vi "observacao.vi"() -> ()   [LabVIEW 2018, in "Shared_160.lvlib"] (continued)
                n2314 = call "TickTimeout.vi"("msInicial"=w2963, "msTimeout"=u32 2000) -> ("msTick"=w2966:u32, "Timeout"=w2965:bool)  [unwired: 1 out]
                n2315 = case shown="True" w2965 {
                  tunnel: w2966 -> [_ w2967]
                  frame False {
                  }
                  frame True {
                    n2316 = global write "Global_Telescopio.vi" "RevCupTO"(w2967) -> ()
                    n2317 = local write "StatDome"("Not Ready" ("Status")) -> ()
                  }
                }
              }
              frame Enabled {
              }
            }
            n2318 = global read "Global_Telescopio.vi" "Senha LEAF"() -> (w2897:string)
            n2319 = call "Bit Status CUP.vi"("NomeStatus"=w2903) -> ("StatBit"=→"trapeiraFechada":bool)
            n2320 = call "Bit Status CUP.vi"("NomeStatus"=w2904) -> ("StatBit"=w2894:bool)
            "trapeiraMovendo" <- w2894
            n2321 = call "Bit Status CUP.vi"("NomeStatus"=w2902) -> ("StatBit"=→"trapeiraAberta":bool)
            n2322 = Not(x=w2894) -> (.not. x?=w2895:bool)
            n2323 = property on="Setup, Pointing & Guiding" class="TabCtl (strict)"("Page Selector Visible"=w2895) -> ()  [unwired: 2 in, 2 out]
            n2324 = Match Pattern(string="OpenShutterPassword", regular expression=w2897) -> (offset past match=w2899:i32)  [unwired: 1 in, 3 out]
            n2325 = Greater Or Equal To 0?(x=w2899) -> (x >= 0?=w2896:bool)
            n2326 = global read "Global_Telescopio.vi" "Telescopio"() -> (w2909:bool)
            n2327 = local read "StatDome"() -> (w2915:string)
            n2328 = Select(t=1, s=w2909, f=2) -> (s? t:f=w2907:i32)
            n2329 = event shown="[3] \"BtShutterOpen\": Value Change" {
              selector: _ -> [_ _ _ _ _ _ _ _]
              dyn-events: _ -> [_ _ _ _ _ _ _ _]
              timeout: 10 -> [_ _ _ _ _ _ _ _]
              tunnel: [FALSE ("NewVal") w3015 w3028 FALSE ("NewVal") FALSE ("NewVal") _ _ _] -> w2913
              tunnel: w2907 -> [_ w3014 _ _ _ _ _ _]
              tunnel: w2896 -> [_ _ _ w3035 _ _ _ _]
              event Timeout {
                n2330 = event-data() -> ()  [unwired: 1 in, 2 out]
              }
              event "BtDomeGO": Value Change {
                n2331 = event-data() -> ("NewVal"=w3016:bool)  [unwired: 1 in, 5 out]
                n2332 = local read "StatDome"() -> (w3019:string)
                n2333 = Equal?(x=w3019, y="Stopped" ("Status")) -> (x = y?=w3017:bool)
                n2334 = And(x=w3016, y=w3017) -> (x .and. y?=w3015:bool)
                n2335 = case shown="True" w3015 {
                  tunnel: w3014 -> [_ w3023]
                  frame False {
                  }
                  frame True {
                    # "20240820"
                    n2336 = local read "DomeNewPos"() -> (w3020:i32)
                    n2337 = Multiply(x=w3020, y=w3023) -> (x*y=w3021:i32)
                    n2338 = call "Checa destino cupula.vi"("Target"=w3021) -> ("moverCup"=w3022:bool)  [unwired: 6 in, 2 out]
                    n2339 = case shown="True" w3022 {
                      tunnel: w3021 -> [_ w3026]
                      frame False {
                      }
                      frame True {
                        # "Desabilita todas Abas"
                        n2340 = local write "DestCUP"(w3026) -> ()
                        n2341 = local write "DOME"(FALSE) -> ()
                        n2342 = property on="Setup, Pointing & Guiding" class="TabCtl (strict)"("Page Selector Visible"=FALSE) -> ()  [unwired: 2 in, 2 out]
                        n2343 = local write "StatDome"("Not Ready" ("Status")) -> ()
                      }
                    }
                  }
                }
              }
              event "BtDomeSTOP": Value Change {
                n2344 = event-data() -> ("NewVal"=w3028:bool)  [unwired: 1 in, 5 out]
                n2345 = case shown="True" w3028 {
                  frame False {
                  }
                  frame True {
                    n2346 = local read "StatDome"() -> (w3029:string)
                    n2347 = case shown="\"Moving\", Default" w3029 {
                      frame "Stopped" {
                      }
                      frame "Moving", Default {
                        w3030 = u16 4 items=["ZERO", "AH", "DEC", "TUBO", "CUP"] ("Controlador")
                        n2348 = local write "StatDome"("Stopping" ("Status")) -> ()
                        n2349 = call "Monta Comando.vi"("Comando"="PARAR", "Dispositivo"="PROG", "Controlador"=w3030) -> ()  [unwired: 2 in, 5 out]
                      }
                      frame "Not Ready" {
                        n2350 = local write "StatDome"("Stopped" ("Status")) -> ()
                      }
                    }
                  }
                }
              }
              event "BtShutterOpen": Value Change {
                # "20250912)"
                n2351 = event-data() -> ("NewVal"=w3038:bool)  [unwired: 1 in, 5 out]
                n2352 = local write "OpenShutterPassword"("") -> ()
                n2353 = And(x=w3038, y=w3035) -> (x .and. y?=w3037:bool)
                n2354 = case shown="True" w3037 {
                  frame False {
                  }
                  frame True {
                    w3040 = FALSE ("WeakSel")
                    w3044 = T5."Enabled" ("Disabled")
                    n2355 = property on="Weak" class="Bool (strict)"("Disabled"=w3044) -> ()  [unwired: 2 in, 2 out]
                    n2356 = local write "Weak"(w3040) -> ()
                    n2357 = local write "WeakSel"(w3040) -> ()
                    n2358 = property on="Medium" class="Bool (strict)"("Disabled"=w3044) -> ()  [unwired: 2 in, 2 out]
                    n2359 = local write "Medium"(w3040) -> ()
                    n2360 = local write "MediumSel"(w3040) -> ()
                    n2361 = call "Log_Shutter.vi"("command"=" ", "domeState"="OPEN " ("command"), "pathLogDomeFile"="C:\\TCS\\LOG\\SHUTTER\\SHUTTER.TXT" ("pathLogFocoString")) -> ()  [unwired: 6 in]
                    n2362 = property on="Strong" class="Bool (strict)"("Disabled"=w3044) -> ()  [unwired: 2 in, 2 out]
                    n2363 = local write "Strong"(w3040) -> ()
                    n2364 = local write "StrongSel"(w3040) -> ()
                    n2365 = stacked-sequence {
                      frame #0 {
                        w3046 = u16 4 items=["ZERO", "AH", "DEC", "TUBO", "CUP"] ("Controlador")
                        n2366 = call "Monta Comando.vi"("Comando"="DESLIGAR", "Dispositivo"="FLAT_WEAK", "Controlador"=w3046) -> ()  [unwired: 2 in, 5 out]
                      }
                      frame #1 {
                        w3049 = u16 4 items=["ZERO", "AH", "DEC", "TUBO", "CUP"] ("Controlador")
                        n2367 = call "Monta Comando.vi"("Comando"="DESLIGAR", "Dispositivo"="FLAT_LO", "Controlador"=w3049) -> ()  [unwired: 2 in, 5 out]
                      }
                      frame #2 {
                        w3052 = u16 4 items=["ZERO", "AH", "DEC", "TUBO", "CUP"] ("Controlador")
                        n2368 = call "Monta Comando.vi"("Comando"="DESLIGAR", "Dispositivo"="FLAT_HI", "Controlador"=w3052) -> ()  [unwired: 2 in, 5 out]
                      }
                      frame #3 {
                        w3054 = u16 4 items=["ZERO", "AH", "DEC", "TUBO", "CUP"] ("Controlador")
                        n2369 = call "Monta Comando.vi"("Comando"="DESLIGAR", "Dispositivo"="FLAT_COUDE", "Controlador"=w3054) -> ()  [unwired: 2 in, 5 out]
                      }
                      frame #4 {
                        w3057 = u16 4 items=["ZERO", "AH", "DEC", "TUBO", "CUP"] ("Controlador")
                        n2370 = call "Monta Comando.vi"("Comando"="ABRIR", "Dispositivo"="TRAPEIRA" ("Comando"), "Controlador"=w3057) -> ()  [unwired: 2 in, 5 out]
                      }
                    }
                    n2371 = property on="Coude" class="Bool (strict)"("DisabledEnum"=w3044) -> ()  [unwired: 2 in, 2 out]
                    n2372 = local write "Coude"(w3040) -> ()
                    n2373 = local write "CoudeSel"(w3040) -> ()
                  }
                }
              }
              event "BtShutterClose": Value Change {
                # "20250912)"
                n2374 = event-data() -> ("NewVal"=w3062:bool)  [unwired: 1 in, 5 out]
                n2375 = local write "OpenShutterPassword"("") -> ()
                n2376 = case shown="True" w3062 {
                  frame False {
                  }
                  frame True {
                    w3064 = u16 4 items=["ZERO", "AH", "DEC", "TUBO", "CUP"] ("Controlador")
                    # "Escreve no LOG o estado do shutter"
                    n2377 = call "Log_Shutter.vi"("command"=" ", "domeState"="CLOSED " ("command"), "pathLogDomeFile"="C:\\TCS\\LOG\\SHUTTER\\SHUTTER.TXT" ("pathLogFocoString")) -> ()  [unwired: 6 in]
                    n2378 = call "Monta Comando.vi"("Comando"="FECHAR", "Dispositivo"="TRAPEIRA" ("Comando"), "Controlador"=w3064) -> ()  [unwired: 2 in, 5 out]
                  }
                }
              }
              event "BtParavUp": Value Change {
                n2379 = event-data() -> ("NewVal"=w3069:bool)  [unwired: 1 in, 5 out]
                n2380 = case shown="True" w3069 {
                  frame False {
                  }
                  frame True {
                    w3072 = u16 4 items=["ZERO", "AH", "DEC", "TUBO", "CUP"] ("Controlador")
                    n2381 = call "Monta Comando.vi"("Comando"="SUBIR", "Dispositivo"="PARAVENTO" ("Comando"), "Controlador"=w3072) -> ()  [unwired: 2 in, 5 out]
                  }
                }
              }
              event "BtParavDown": Value Change {
                n2382 = event-data() -> ("NewVal"=w3073:bool)  [unwired: 1 in, 5 out]
                n2383 = case shown="True" w3073 {
                  frame False {
                  }
                  frame True {
                    w3076 = u16 4 items=["ZERO", "AH", "DEC", "TUBO", "CUP"] ("Controlador")
                    n2384 = call "Monta Comando.vi"("Comando"="DESCER", "Dispositivo"="PARAVENTO" ("Comando"), "Controlador"=w3076) -> ()  [unwired: 2 in, 5 out]
                  }
                }
              }
              event "BtParavStop": Value Change {
                n2385 = event-data() -> ("NewVal"=w3077:bool)  [unwired: 1 in, 5 out]
                n2386 = case shown="True" w3077 {
                  frame False {
                  }
                  frame True {
                    w3080 = u16 4 items=["ZERO", "AH", "DEC", "TUBO", "CUP"] ("Controlador")
                    n2387 = call "Monta Comando.vi"("Comando"="PARAR", "Dispositivo"="PARAVENTO" ("Comando"), "Controlador"=w3080) -> ()  [unwired: 2 in, 5 out]
                  }
                }
              }
            }
            n2388 = call "Bit Status CUP.vi"("NomeStatus"=w2914) -> ("StatBit"=w2912:bool)
            n2389 = global read "Global_Telescopio.vi" "PosCUP"() -> (w2911:i16)
            n2390 = case shown="\"Not Ready\"" w2915 {
              tunnel: w2912 -> [_ _ w3004 w3010]
              tunnel: w2913 -> [_ _ _ _]
              frame "", Default {
              }
              frame "Not Ready" {
                n2391 = local read "DestCUP"() -> (w2990:i16)
                n2392 = global read "Global_Telescopio.vi" "PosCUP"() -> (w2992:i16)
                n2393 = call "TickTimeout.vi"() -> ("msTick"=w2993:u32)  [unwired: 2 in, 2 out]
                n2394 = call "Checa destino cupula.vi"("Target"=w2990) -> ("moverCup"=w2989:bool, "angTarget"=w2991:string)  [unwired: 6 in, 1 out]
                n2395 = case shown="True" w2989 {
                  tunnel: w2993 -> [_ w2999]
                  tunnel: w2992 -> [_ w2998]
                  tunnel: w2991 -> [_ w2997]
                  tunnel: w2990 -> [_ w2996]
                  frame False {
                    n2396 = local write "StatDome"("Stopping" ("Status")) -> ()
                  }
                  frame True {
                    w3003 = u16 4 items=["ZERO", "AH", "DEC", "TUBO", "CUP"] ("Controlador")
                    # "20240820"
                    n2397 = global write "Global_Telescopio.vi" "RevCupTO"(w2999) -> ()
                    n2398 = local write "TargetCup"(w2997) -> ()
                    n2399 = global write "Global_Telescopio.vi" "CupStartPos"(w2998) -> ()
                    n2400 = Number To Decimal String(number=w2996) -> (decimal integer string=w3000:string)  [unwired: 1 in]
                    n2401 = local write "StatDome"("Moving" ("Status")) -> ()
                    n2402 = call "Monta Comando.vi"("Set Point"=w3000, "Comando"="MOVER", "Dispositivo"="DOMO" ("Comando"), "Controlador"=w3003) -> ()  [unwired: 1 in, 5 out]
                  }
                }
              }
              frame "Moving" {
                n2403 = case shown="False" w3004 {
                  frame False {
                    n2404 = local read "DestCUP"() -> (w3009:i16)
                    n2405 = call "Checa destino cupula.vi"("Target"=w3009) -> ("moverCup"=w3008:bool)  [unwired: 6 in, 2 out]
                    n2406 = Select(t="Not Ready" ("Comando"), s=w3008, f="Stopping" ("Comando")) -> (s? t:f=w3007:string)
                    n2407 = local write "StatDome"(w3007) -> ()
                  }
                  frame True {
                  }
                }
              }
              frame "Stopping" {
                n2408 = case shown="False" w3010 {
                  frame False {
                    # "Reabilita Abas"
                    n2409 = property on="Setup, Pointing & Guiding" class="TabCtl (strict)"("Page Selector Visible"=TRUE) -> ()  [unwired: 2 in, 2 out]
                    n2410 = local write "StatDome"("Stopped" ("Status")) -> ()
                  }
                  frame True {
                  }
                }
              }
            }
            n2411 = Divide(x=w2911, y=w2907) -> (x/y=w2918:dbl)
            n2412 = To Word Integer(number=w2918) -> (16bit integer=→"AngCup":i16)
            n2413 = event shown="[4] \"CW\": Mouse Up" {
              selector: _ -> [_ _ _ _ _]
              dyn-events: _ -> [_ _ _ _ _]
              timeout: 100 -> [_ _ _ _ _]
              event Timeout {
                n2414 = event-data() -> ()  [unwired: 1 in, 2 out]
              }
              event "CCW": Mouse Down {
                w2969 = "GIRAR_CCW" ("Comando")
                w2970 = u16 4 items=["ZERO", "AH", "DEC", "TUBO", "CUP"] ("Controlador")
                # "Envia o comando GIRAR"
                n2415 = event-data() -> ()  [unwired: 1 in, 7 out]
                n2416 = local write "Command"(w2969) -> ()
                n2417 = call "Monta Comando.vi"("Comando"=w2969, "Dispositivo"="DOMO" ("Comando"), "Controlador"=w2970) -> ()  [unwired: 2 in, 5 out]
              }
              event "CCW": Mouse Up {
                n2418 = event-data() -> ()  [unwired: 1 in, 7 out]
                n2419 = stacked-sequence {
                  frame #0 {
                    w2972 = "PARAR" ("Comando")
                    w2973 = u16 4 items=["ZERO", "AH", "DEC", "TUBO", "CUP"] ("Controlador")
                    # "Envia o comando PARAR"
                    n2420 = local write "Command"(w2972) -> ()
                    n2421 = call "Monta Comando.vi"("Comando"=w2972, "Dispositivo"="DOMO" ("Comando"), "Controlador"=w2973) -> ()  [unwired: 2 in, 5 out]
                  }
                  frame #1 {
                    n2422 = Wait (ms)(milliseconds to wait=u32 100) -> ()  [unwired: 1 out]
                  }
                  frame #2 {
                    w2976 = "PARAR" ("Comando")
                    w2977 = u16 4 items=["ZERO", "AH", "DEC", "TUBO", "CUP"] ("Controlador")
                    # "Envia o comando PARAR"
                    n2423 = local write "Command"(w2976) -> ()
                    n2424 = call "Monta Comando.vi"("Comando"=w2976, "Dispositivo"="DOMO" ("Comando"), "Controlador"=w2977) -> ()  [unwired: 2 in, 5 out]
                  }
                }
              }
              event "CW": Mouse Down {
                w2979 = "GIRAR_CW" ("Comando")
                w2980 = u16 4 items=["ZERO", "AH", "DEC", "TUBO", "CUP"] ("Controlador")
                # "Envia o comando GIRAR"
                n2425 = event-data() -> ()  [unwired: 1 in, 7 out]
                n2426 = local write "Command"(w2979) -> ()
                n2427 = call "Monta Comando.vi"("Comando"=w2979, "Dispositivo"="DOMO" ("Comando"), "Controlador"=w2980) -> ()  [unwired: 2 in, 5 out]
              }
              event "CW": Mouse Up {
                n2428 = event-data() -> ()  [unwired: 1 in, 7 out]
                n2429 = stacked-sequence {
                  frame #0 {
                    w2982 = "PARAR" ("Comando")
                    w2983 = u16 4 items=["ZERO", "AH", "DEC", "TUBO", "CUP"] ("Controlador")
                    # "Envia o comando PARAR"
                    n2430 = local write "Command"(w2982) -> ()
                    n2431 = call "Monta Comando.vi"("Comando"=w2982, "Dispositivo"="DOMO" ("Comando"), "Controlador"=w2983) -> ()  [unwired: 2 in, 5 out]
                  }
                  frame #1 {
                    n2432 = Wait (ms)(milliseconds to wait=u32 100) -> ()  [unwired: 1 out]
                  }
                  frame #2 {
                    w2986 = "PARAR" ("Comando")
                    w2987 = u16 4 items=["ZERO", "AH", "DEC", "TUBO", "CUP"] ("Controlador")
                    # "Envia o comando PARAR"
                    n2433 = local write "Command"(w2986) -> ()
                    n2434 = call "Monta Comando.vi"("Comando"=w2986, "Dispositivo"="DOMO" ("Comando"), "Controlador"=w2987) -> ()  [unwired: 2 in, 5 out]
                  }
                }
              }
            }
            "Command" <- "" ("Command")
          }
          frame "UTILS " {
            n2435 = stacked-sequence {
              frame #0 {
                # "Acionamento das Abas do\nEspelho\n\nComandos sempre precedidos\nde ESPAÇO\n\nTUBO TAMPAS ESCREVER = 80 80\n\nLigar power geral       08 08\nDesligar power geral  08 00\nLigar System              10 10\nDesligar System         10 00\nPassar para Remoto  20 20\nPassar para Local      20 00\nSel. device central     40 40\nSel. device bowl         40 00\nAction open                80 80\nAction close                80 00"
                n2436 = event shown="[1] \"MODE\": Value Change" {
                  selector: _ -> [_ _ _]
                  dyn-events: _ -> [_ _ _]
                  timeout: 10 -> [_ _ _]
                  event Timeout {
                    n2437 = event-data() -> ()  [unwired: 1 in, 2 out]
                  }
                  event "MODE": Value Change {
                    n2438 = event-data() -> ("NewVal"=w3095:bool)  [unwired: 1 in, 5 out]
                    "LED MODE" <- w3095
                    n2439 = case shown="False" w3095 {
                      frame False {
                        w3100 = u16 3 items=["ZERO", "AH", "DEC", "TUBO", "CUP"] ("Controlador")
                        # "DESABILITA"
                        # "APENAS PASSANDO COMANDO PARA MANETE"
                        # "MODE E GERAL = 0"
                        # "MODE HADSET"
                        n2440 = call "Monta Comando.vi"("Set Point"=" F8 90", "Comando"="ESCREVER", "Dispositivo"="TAMPAS" ("Comando"), "Controlador"=w3100) -> ()  [unwired: 1 in, 5 out]
                        n2441 = property on="ACTION" class="Bool (strict)"("Disabled"=u8 2) -> ()  [unwired: 2 in, 2 out]
                      }
                      frame True {
                        w3105 = u16 3 items=["ZERO", "AH", "DEC", "TUBO", "CUP"] ("Controlador")
                        # "HABILITA"
                        # "APENAS PASSANDO COMOANDO PARA TCSPD"
                        # "MODE E GERAL = 1"
                        # "MODE TCSPD"
                        n2442 = call "Monta Comando.vi"("Set Point"=" 48 48", "Comando"="ESCREVER", "Dispositivo"="TAMPAS" ("Comando"), "Controlador"=w3105) -> ()  [unwired: 1 in, 5 out]
                        n2443 = property on="ACTION" class="Bool (strict)"("Disabled"=u8 0) -> ()  [unwired: 2 in, 2 out]
                      }
                    }
                  }
                  event "ACTION": Value Change {
                    n2444 = event-data() -> ("NewVal"=w3106:bool)  [unwired: 1 in, 5 out]
                    n2445 = case shown="False" w3106 {
                      frame False {
                        # "FECHAR"
                        n2446 = local write "ESTADO FECHAR"("INICIO" ("ESTADO ABRIR")) -> ()
                        n2447 = local write "ESTADO ABRIR"("REPOUSO" ("ESTADO ABRIR")) -> ()
                      }
                      frame True {
                        # "ABRIR"
                        n2448 = local write "ESTADO FECHAR"("REPOUSO" ("ESTADO ABRIR")) -> ()
                        n2449 = local write "ESTADO ABRIR"("INICIO" ("ESTADO ABRIR")) -> ()
                      }
                    }
                  }
                }
                n2450 = Tick Count (ms)() -> (millisecond timer value=w3086:u32)
                n2451 = Greater Or Equal?(x=w3086, y="TIMER TICK") -> (x >= y?=w3082:bool)
                n2452 = And(x=w3082, y=FALSE) -> (x .and. y?=w3083:bool)
                n2453 = case shown="True" w3083 {
                  frame False {
                  }
                  frame True {
                    w3119 = u16 3 items=["ZERO", "AH", "DEC", "TUBO", "CUP", "CASS", "COUDE"] ("Controlador")
                    # "2 SEGUNDOS"
                    n2454 = Tick Count (ms)() -> (millisecond timer value=w3116:u32)
                    n2455 = Add(x=w3116, y=u32 10000) -> (x+y=w3114:u32)
                    n2456 = call "Status_das_Tampas.vi"("Controlador"=w3119, "DISPOSITIVO"="TAMPAS", "Comando"="LER") -> ("Fechado/Aberto"=w3113:bool, "Dispositivo Bacia/Centar"=w3112:bool)  [unwired: 6 in, 5 out]
                    n2457 = local write "TIMER TICK"(w3114) -> ()
                    n2458 = Not(x=w3113) -> (.not. x?=w3111:bool)
                    n2459 = And(x=w3111, y=w3112) -> ()  [unwired: 1 out]
                  }
                }
                n2460 = event shown="[4] \"FLAT-FIELD\": Value Change" {
                  selector: _ -> [_ _ _ _ _ _]
                  dyn-events: _ -> [_ _ _ _ _ _]
                  timeout: 10 -> [_ _ _ _ _ _]
                  event Timeout {
                    n2461 = event-data() -> ()  [unwired: 1 in, 2 out]
                  }
                  event "BtUtilPark": Value Change {
                    n2462 = event-data() -> ("NewVal"=w3120:bool)  [unwired: 1 in, 5 out]
                    n2463 = case shown="True" w3120 {
                      frame False {
                      }
                      frame True {
                        w3123 = u16 4 items=["ZERO", "AH", "DEC", "TUBO", "CUP"] ("Controlador")
                        w3124 = FALSE ("MOUNT")
                        w3127 = 0 ("M_AH")
                        w3128 = u8 2 ("Disabled")
                        w3125 = FALSE ("Page Selector Visible")
                        w3132 = 1 ("M_AH")
                        # "Carrega Parâmetros da Configuração"
                        # "Seta Máq GO"
                        # "Desabilita todas Abas"
                        # "DESABILITA TODOS"
                        n2464 = local write "DOME"(w3125) -> ()
                        n2465 = property on="Setup, Pointing & Guiding" class="TabCtl (strict)"("Page Selector Visible"=w3125) -> ()  [unwired: 2 in, 2 out]
                        n2466 = local write "statAH"(w3127) -> ()
                        n2467 = local write "statCUP"(w3127) -> ()
                        n2468 = local write "statDEC"(w3127) -> ()
                        n2469 = local write "M_DEC"(w3132) -> ()
                        n2470 = local write "M_AH"(w3132) -> ()
                        n2471 = local write "M_CUP"(w3132) -> ()
                        n2472 = global read "Global_Telescopio.vi" "DestDEC"() -> (w3130:dbl)
                        n2473 = global read "Global_Telescopio.vi" "DestCUP"() -> (w3129:i32)
                        n2474 = global read "Global_Telescopio.vi" "DestAH"() -> (w3131:dbl)
                        n2475 = property on="BtUtilPark" class="Bool (strict)"("Disabled"=w3128) -> ()  [unwired: 2 in, 2 out]
                        n2476 = property on="ECASS" class="Bool (strict)"("Disabled"=w3128) -> ()  [unwired: 2 in, 2 out]
                        n2477 = local write "DestAH"(w3131) -> ()
                        n2478 = local write "DestCUP"(w3129) -> ()
                        n2479 = local write "DestDEC"(w3130) -> ()
                        n2480 = global write "Global_Telescopio.vi" "Parking"(TRUE ("Page Selector Visible")) -> ()
                        n2481 = property on="BtUtilZenith" class="Bool (strict)"("Disabled"=w3128) -> ()  [unwired: 2 in, 2 out]
                        n2482 = property on="FLAT-FIELD" class="Bool (strict)"("Disabled"=w3128) -> ()  [unwired: 2 in, 2 out]
                        n2483 = property on="PROTEÇÃO" class="Bool (strict)"("Disabled"=w3128) -> ()  [unwired: 2 in, 2 out]
                        n2484 = local write "MOUNT"(w3124) -> ()
                        n2485 = local write "GUIDER"(w3124) -> ()
                        n2486 = call "Monta Comando.vi"("Comando"="LIGAR", "Dispositivo"="LAMP_CAM" ("Comando"), "Controlador"=w3123) -> ()  [unwired: 2 in, 5 out]
                      }
                    }
                  }
                  event "BtUtilZenith": Value Change {
                    n2487 = event-data() -> ("NewVal"=w3133:bool)  [unwired: 1 in, 5 out]
                    n2488 = case shown="True" w3133 {
                      frame False {
                      }
                      frame True {
                        w3136 = u16 4 items=["ZERO", "AH", "DEC", "TUBO", "CUP"] ("Controlador")
                        w3137 = FALSE ("MOUNT")
                        w3140 = 0 ("M_AH")
                        w3141 = u8 2 ("Disabled")
                        w3139 = FALSE ("Page Selector Visible")
                        w3145 = 1 ("M_AH")
                        # "Seta Máq GO"
                        # "Desabilita todas Abas"
                        # "DESABILITA TODOS"
                        n2489 = local write "M_DEC"(w3145) -> ()
                        n2490 = local write "M_AH"(w3145) -> ()
                        n2491 = local write "M_CUP"(w3145) -> ()
                        n2492 = local write "DOME"(w3139) -> ()
                        n2493 = property on="Setup, Pointing & Guiding" class="TabCtl (strict)"("Page Selector Visible"=w3139) -> ()  [unwired: 2 in, 2 out]
                        n2494 = call "Monta Comando.vi"("Comando"="LIGAR", "Dispositivo"="LAMP_CAM" ("Comando"), "Controlador"=w3136) -> ()  [unwired: 2 in, 5 out]
                        n2495 = local write "statAH"(w3140) -> ()
                        n2496 = local write "statCUP"(w3140) -> ()
                        n2497 = local write "statDEC"(w3140) -> ()
                        n2498 = global read "Global_Telescopio.vi" "Telescopio"() -> (w3138:bool)
                        n2499 = property on="BtUtilPark" class="Bool (strict)"("Disabled"=w3141) -> ()  [unwired: 2 in, 2 out]
                        n2500 = property on="ECASS" class="Bool (strict)"("Disabled"=w3141) -> ()  [unwired: 2 in, 2 out]
                        n2501 = case shown="False" w3138 {
                          tunnel: [0.0 ("DestAH") 0.0 ("DestAH")] -> w3144
                          tunnel: [-0.3933 ("DestDEC") -0.3933 ("DestDEC")] -> w3143
                          tunnel: [i16 98 ("DestCUP") i16 80 ("DestCUP")] -> w3142
                          frame False {
                          }
                          frame True {
                          }
                        }
                        n2502 = property on="BtUtilZenith" class="Bool (strict)"("Disabled"=w3141) -> ()  [unwired: 2 in, 2 out]
                        n2503 = property on="FLAT-FIELD" class="Bool (strict)"("Disabled"=w3141) -> ()  [unwired: 2 in, 2 out]
                        n2504 = local write "DestAH"(w3144) -> ()
                        n2505 = local write "DestCUP"(w3142) -> ()
                        n2506 = local write "DestDEC"(w3143) -> ()
                        n2507 = property on="PROTEÇÃO" class="Bool (strict)"("Disabled"=w3141) -> ()  [unwired: 2 in, 2 out]
                        n2508 = local write "MOUNT"(w3137) -> ()
                        n2509 = local write "GUIDER"(w3137) -> ()
                      }
                    }
                  }
                  event "ECASS": Value Change {
                    n2510 = event-data() -> ("NewVal"=w3152:bool)  [unwired: 1 in, 5 out]
                    n2511 = case shown="True" w3152 {
                      frame False {
                      }
                      frame True {
                        w3155 = u16 4 items=["ZERO", "AH", "DEC", "TUBO", "CUP"] ("Controlador")
                        w3156 = FALSE ("MOUNT")
                        w3159 = 0 ("M_AH")
                        w3160 = u8 2 ("Disabled")
                        w3158 = FALSE ("Page Selector Visible")
                        w3164 = 1 ("M_AH")
                        # "Seta Máq GO"
                        # "Desabilita todas Abas"
                        # "DESABILITA TODOS"
                        n2512 = local write "M_DEC"(w3164) -> ()
                        n2513 = local write "M_AH"(w3164) -> ()
                        n2514 = local write "M_CUP"(w3164) -> ()
                        n2515 = local write "DOME"(w3158) -> ()
                        n2516 = property on="Setup, Pointing & Guiding" class="TabCtl (strict)"("Page Selector Visible"=w3158) -> ()  [unwired: 2 in, 2 out]
                        n2517 = local write "statAH"(w3159) -> ()
                        n2518 = local write "statCUP"(w3159) -> ()
                        n2519 = local write "statDEC"(w3159) -> ()
                        n2520 = call "Monta Comando.vi"("Comando"="LIGAR", "Dispositivo"="LAMP_CAM" ("Comando"), "Controlador"=w3155) -> ()  [unwired: 2 in, 5 out]
                        n2521 = global read "Global_Telescopio.vi" "Telescopio"() -> (w3157:bool)
                        n2522 = property on="BtUtilPark" class="Bool (strict)"("Disabled"=w3160) -> ()  [unwired: 2 in, 2 out]
                        n2523 = property on="ECASS" class="Bool (strict)"("Disabled"=w3160) -> ()  [unwired: 2 in, 2 out]
                        n2524 = property on="BtUtilZenith" class="Bool (strict)"("Disabled"=w3160) -> ()  [unwired: 2 in, 2 out]
                        n2525 = property on="FLAT-FIELD" class="Bool (strict)"("Disabled"=w3160) -> ()  [unwired: 2 in, 2 out]
                        n2526 = case shown="False" w3157 {
                          tunnel: [0.0 ("DestAH") 0.0 ("DestAH")] -> w3163
                          tunnel: [0.4 ("DestDEC") 0.4 ("DestDEC")] -> w3162
                          tunnel: [i16 98 ("DestCUP") i16 80 ("DestCUP")] -> w3161
                          frame False {
                          }
                          frame True {
                          }
                        }
                        n2527 = property on="PROTEÇÃO" class="Bool (strict)"("Disabled"=w3160) -> ()  [unwired: 2 in, 2 out]
                        n2528 = local write "MOUNT"(w3156) -> ()
                        n2529 = local write "GUIDER"(w3156) -> ()
                        n2530 = local write "DestAH"(w3163) -> ()
                        n2531 = local write "DestCUP"(w3161) -> ()
                        n2532 = local write "DestDEC"(w3162) -> ()
                      }
                    }
                  }
                  event "FLAT-FIELD": Value Change {
                    n2533 = event-data() -> ("NewVal"=w3171:bool)  [unwired: 1 in, 5 out]
                    n2534 = case shown="True" w3171 {
                      frame False {
                      }
                      frame True {
                        w3174 = u16 4 items=["ZERO", "AH", "DEC", "TUBO", "CUP"] ("Controlador")
                        w3175 = FALSE ("MOUNT")
                        w3177 = 0 ("M_AH")
                        w3179 = u8 2 ("Disabled")
                        w3178 = FALSE ("Page Selector Visible")
                        w3183 = 1 ("M_AH")
                        # "Seta Máq GO"
                        # "Desabilita todas Abas"
                        # "DESABILITA TODOS"
                        n2535 = local write "M_DEC"(w3183) -> ()
                        n2536 = local write "M_AH"(w3183) -> ()
                        n2537 = local write "M_CUP"(w3183) -> ()
                        n2538 = local write "DOME"(w3178) -> ()
                        n2539 = property on="Setup, Pointing & Guiding" class="TabCtl (strict)"("Page Selector Visible"=w3178) -> ()  [unwired: 2 in, 2 out]
                        n2540 = call "Monta Comando.vi"("Comando"="LIGAR", "Dispositivo"="LAMP_CAM" ("Comando"), "Controlador"=w3174) -> ()  [unwired: 2 in, 5 out]
                        n2541 = local write "statAH"(w3177) -> ()
                        n2542 = local write "statCUP"(w3177) -> ()
                        n2543 = local write "statDEC"(w3177) -> ()
                        n2544 = global read "Global_Telescopio.vi" "Telescopio"() -> (w3176:bool)
                        n2545 = property on="BtUtilPark" class="Bool (strict)"("Disabled"=w3179) -> ()  [unwired: 2 in, 2 out]
                        n2546 = property on="ECASS" class="Bool (strict)"("Disabled"=w3179) -> ()  [unwired: 2 in, 2 out]
                        n2547 = case shown="False" w3176 {
                          tunnel: [0.0715 ("DestAH") 0.31416 ("DestAH")] -> w3182
                          tunnel: [0.641 ("DestDEC") -0.39415 ("DestDEC")] -> w3181
                          tunnel: [i16 306 ("DestCUP") i16 133 ("DestCUP")] -> w3180
                          frame False {
                          }
                          frame True {
                          }
                        }
                        n2548 = property on="BtUtilZenith" class="Bool (strict)"("Disabled"=w3179) -> ()  [unwired: 2 in, 2 out]
                        n2549 = property on="FLAT-FIELD" class="Bool (strict)"("Disabled"=w3179) -> ()  [unwired: 2 in, 2 out]
                        n2550 = local write "DestAH"(w3182) -> ()
                        n2551 = local write "DestCUP"(w3180) -> ()
                        n2552 = local write "DestDEC"(w3181) -> ()
                        n2553 = property on="PROTEÇÃO" class="Bool (strict)"("Disabled"=w3179) -> ()  [unwired: 2 in, 2 out]
                        n2554 = local write "GUIDER"(w3175) -> ()
                        n2555 = local write "MOUNT"(w3175) -> ()
                      }
                    }
                  }
                  event "PROTEÇÃO": Value Change {
                    n2556 = event-data() -> ("NewVal"=w3190:bool)  [unwired: 1 in, 5 out]
                    n2557 = case shown="True" w3190 {
                      frame False {
                      }
                      frame True {
                        w3191 = FALSE ("MOUNT")
                        w3193 = 0 ("M_AH")
                        w3192 = FALSE ("Page Selector Visible")
                        w3195 = u8 2 ("Disabled")
                        # "Seta Máq GO"
                        # "Desabilita todas Abas"
                        # "DESABILITA TODOS"
                        n2558 = local write "DOME"(w3192) -> ()
                        n2559 = property on="Setup, Pointing & Guiding" class="TabCtl (strict)"("Page Selector Visible"=w3192) -> ()  [unwired: 2 in, 2 out]
                        n2560 = local write "statAH"(w3193) -> ()
                        n2561 = local write "statCUP"(w3193) -> ()
                        n2562 = local write "statDEC"(w3193) -> ()
                        n2563 = property on="BtUtilPark" class="Bool (strict)"("Disabled"=w3195) -> ()  [unwired: 2 in, 2 out]
                        n2564 = property on="ECASS" class="Bool (strict)"("Disabled"=w3195) -> ()  [unwired: 2 in, 2 out]
                        n2565 = property on="BtUtilZenith" class="Bool (strict)"("Disabled"=w3195) -> ()  [unwired: 2 in, 2 out]
                        n2566 = property on="FLAT-FIELD" class="Bool (strict)"("Disabled"=w3195) -> ()  [unwired: 2 in, 2 out]
                        n2567 = local write "M_PROT"(1 ("M_PROT")) -> ()
                        n2568 = local write "MOUNT"(w3191) -> ()
                        n2569 = local write "GUIDER"(w3191) -> ()
                        n2570 = property on="PROTEÇÃO" class="Bool (strict)"("Disabled"=w3195) -> ()  [unwired: 2 in, 2 out]
                      }
                    }
                  }
                }
                n2571 = case shown="True" "STOP" {
                  frame False {
                  }
                  frame True {
                    n2572 = stacked-sequence {
                      frame #0 {
                        w3197 = 0 ("estado")
                        # "Zera Máquina de Estado\nPelo Botão STOP"
                        n2573 = property on="Setup, Pointing & Guiding" class="TabCtl (strict)"("Page Selector Visible"=TRUE) -> ()  [unwired: 2 in, 2 out]
                        n2574 = call "Stop.vi"() -> ()  [unwired: 1 in, 1 out]
                        n2575 = local write "Flag Stop"(TRUE ("Flag Stop")) -> ()
                        n2576 = local write "M_AH"(w3197) -> ()
                        n2577 = local write "M_DEC"(w3197) -> ()
                        n2578 = local write "M_CUP"(w3197) -> ()
                        n2579 = local write "M_PROT"(w3197) -> ()
                      }
                      frame #1 {
                        w3199 = FALSE
                        w3200 = u8 0 ("Disabled")
                        # "DESLIGA TODOS"
                        # "HABILITA TODOS"
                        n2580 = local write "BtUtilZenith"(w3199) -> ()
                        n2581 = local write "BtUtilPark"(w3199) -> ()
                        n2582 = local write "FLAT-FIELD"(w3199) -> ()
                        n2583 = local write "PROTEÇÃO"(w3199) -> ()
                        n2584 = local write "ECASS"(w3199) -> ()
                        n2585 = property on="BtUtilPark" class="Bool (strict)"("Disabled"=w3200) -> ()  [unwired: 2 in, 2 out]
                        n2586 = property on="ECASS" class="Bool (strict)"("Disabled"=w3200) -> ()  [unwired: 2 in, 2 out]
                        n2587 = property on="BtUtilZenith" class="Bool (strict)"("Disabled"=w3200) -> ()  [unwired: 2 in, 2 out]
                        n2588 = property on="PROTEÇÃO" class="Bool (strict)"("Disabled"=w3200) -> ()  [unwired: 2 in, 2 out]
                        n2589 = property on="FLAT-FIELD" class="Bool (strict)"("Disabled"=w3200) -> ()  [unwired: 2 in, 2 out]
                      }
                    }
                  }
                }
                n2590 = Compound Arithmetic op=OR("BtUtilPark", "BtUtilZenith", "ECASS", "FLAT-FIELD", "PROTEÇÃO") -> (→"MOVING":bool)
              }
              frame #1 {
                # "MÁQUINAS DE ESTADOS DAS TAMPAS"
                n2591 = case shown="True" "Case Constant\n(See Context Help) 11" {
                  frame False {
                    # "ABRIR"
                    # "FECHAR"
                    n2592 = case shown="\"PIZZA\"" "ESTADO FECHAR" {
                      tunnel: [w3251 w3259 w3270 w3278 w3288 w3296 w3306 "REPOUSO" ("y")] -> w3205
                      frame "INICIO", Default {
                        w3256 = u16 3 items=["ZERO", "AH", "DEC", "TUBO", "CUP"] ("Controlador")
                        # "SELECIONA DISPOSITVO BACIA E\nMANDA FECHAR"
                        # "DISP=1 E PIZZA=1"
                        n2593 = call "Monta Comando.vi"("Set Point"=" A0 A0", "Comando"="ESCREVER", "Dispositivo"="TAMPAS" ("Comando"), "Controlador"=w3256) -> ("Resposta"=w3252:string)  [unwired: 1 in, 4 out]
                        n2594 = Not Equal?(x=w3252, y="TAMPAS OK") -> ()  [unwired: 1 out]
                        n2595 = Tick Count (ms)() -> (millisecond timer value=→"T1 2":u32)
                        n2596 = Select(t="REPOUSO" ("y"), s=FALSE, f="ESPERA 1" ("y")) -> (s? t:f=w3251:string)
                      }
                      frame "ESPERA 1" {
                        # "20 SEGUNDOS"
                        n2597 = local read "T1 2"() -> (w3264:u32)
                        n2598 = Tick Count (ms)() -> (millisecond timer value=w3262:u32)
                        n2599 = Add(x=w3264, y=u32 20000) -> (x+y=w3261:u32)
                        n2600 = Greater?(x=w3262, y=w3261) -> (0:w3258:bool)
                        n2601 = Select(t="PIZZA" ("y"), s=w3258, f="ESPERA 1" ("y")) -> (s? t:f=w3259:string)
                      }
                      frame "PIZZA" {
                        w3275 = u16 3 items=["ZERO", "AH", "DEC", "TUBO", "CUP"] ("Controlador")
                        # "SELECIONA DISP PIZZA\nE MANDA FECHAR"
                        # "PIZZA=1"
                        n2602 = call "Monta Comando.vi"("Set Point"=" 30 10", "Comando"="ESCREVER", "Dispositivo"="TAMPAS" ("Comando"), "Controlador"=w3275) -> ("Resposta"=w3269:string)  [unwired: 1 in, 4 out]
                        n2603 = Tick Count (ms)() -> (millisecond timer value=→"T2 2":u32)
                        n2604 = Not Equal?(x=w3269, y="TAMPAS OK") -> ()  [unwired: 1 out]
                        n2605 = Select(t="REPOUSO" ("y"), s=FALSE, f="PIZZA 2") -> (s? t:f=w3270:string)
                      }
                      frame "PIZZA 2" {
                        w3286 = u16 3 items=["ZERO", "AH", "DEC", "TUBO", "CUP"] ("Controlador")
                        n2606 = call "Monta Comando.vi"("Set Point"=" F8 90", "Comando"="ESCREVER", "Dispositivo"="TAMPAS" ("Comando"), "Controlador"=w3286) -> ("Resposta"=w3281:string)  [unwired: 1 in, 4 out]
                        n2607 = Tick Count (ms)() -> (millisecond timer value=→"T2 3":u32)
                        n2608 = Not Equal?(x=w3281, y="TAMPAS OK") -> ()  [unwired: 1 out]
                        n2609 = Select(t="REPOUSO" ("y"), s=FALSE, f="ESPERA 1A") -> (s? t:f=w3278:string)
                      }
                      frame "ESPERA 1A" {
                        # "2 SEGUNDOS"
                        n2610 = local read "T2 3"() -> (w3291:u32)
                        n2611 = Tick Count (ms)() -> (millisecond timer value=w3293:u32)
                        n2612 = Add(x=w3291, y=u32 2000) -> (x+y=w3294:u32)
                        n2613 = Greater?(x=w3293, y=w3294) -> (0:w3287:bool)
                        n2614 = Select(t="PIZZA 3" ("y"), s=w3287, f="ESPERA 1A" ("y")) -> (s? t:f=w3288:string)
                      }
                      frame "PIZZA 3" {
                        w3304 = u16 3 items=["ZERO", "AH", "DEC", "TUBO", "CUP"] ("Controlador")
                        # "PIZZA=3"
                        n2615 = call "Monta Comando.vi"("Set Point"=" 48 48", "Comando"="ESCREVER", "Dispositivo"="TAMPAS" ("Comando"), "Controlador"=w3304) -> ("Resposta"=w3299:string)  [unwired: 1 in, 4 out]
                        n2616 = Not Equal?(x=w3299, y="TAMPAS OK") -> ()  [unwired: 1 out]
                        n2617 = Select(t="REPOUSO" ("y"), s=FALSE, f="ESPERA 2" ("y")) -> (s? t:f=w3296:string)
                      }
                      frame "ESPERA 2" {
                        # "10 SEGUNDOS"
                        n2618 = local read "T2 2"() -> (w3310:u32)
                        n2619 = Tick Count (ms)() -> (millisecond timer value=w3308:u32)
                        n2620 = Add(x=w3310, y=u32 10000) -> (x+y=w3307:u32)
                        n2621 = Greater?(x=w3308, y=w3307) -> (0:w3305:bool)
                        n2622 = case shown="True" w3305 {
                          frame False {
                          }
                          frame True {
                            n2623 = local write "LED ACTION"(FALSE ("LED ACTION")) -> ()
                          }
                        }
                        n2624 = Select(t="REPOUSO" ("y"), s=w3305, f="ESPERA 2" ("y")) -> (s? t:f=w3306:string)
                      }
                      frame "REPOUSO" {
                      }
                    }
                    n2625 = local write "ESTADO FECHAR"(w3205) -> ()
                    n2626 = case shown="\"INICIO\", Default" "ESTADO ABRIR" {
                      tunnel: [w3210 w3219 w3230 w3237 "REPOUSO" ("y")] -> w3203
                      frame "INICIO", Default {
                        w3216 = u16 3 items=["ZERO", "AH", "DEC", "TUBO", "CUP"] ("Controlador")
                        # "SELECIONA DISPOSITVO PIZZA E\nMANDA ABRIR"
                        # "DISP=0 E PIZZA=0"
                        n2627 = call "Monta Comando.vi"("Set Point"=" 30 00", "Comando"="ESCREVER", "Dispositivo"="TAMPAS" ("Comando"), "Controlador"=w3216) -> ("Resposta"=w3211:string)  [unwired: 1 in, 4 out]
                        n2628 = Not Equal?(x=w3211, y="TAMPAS OK") -> ()  [unwired: 1 out]
                        n2629 = Tick Count (ms)() -> (millisecond timer value=→"T1":u32)
                        n2630 = Select(t="REPOUSO" ("y"), s=FALSE, f="ESPERA 1" ("y")) -> (s? t:f=w3210:string)
                      }
                      frame "ESPERA 1" {
                        # "10 SEGUNDOS"
                        n2631 = local read "T1"() -> (w3224:u32)
                        n2632 = Tick Count (ms)() -> (millisecond timer value=w3222:u32)
                        n2633 = Add(x=w3224, y=u32 10000) -> (x+y=w3221:u32)
                        n2634 = Greater?(x=w3222, y=w3221) -> (0:w3218:bool)
                        n2635 = Select(t="BACIA" ("y"), s=w3218, f="ESPERA 1" ("y")) -> (s? t:f=w3219:string)
                      }
                      frame "BACIA" {
                        w3235 = u16 3 items=["ZERO", "AH", "DEC", "TUBO", "CUP"] ("Controlador")
                        # "SELECIONA DISP BACIA\nE MANDA ABRIR"
                        # "BACIA=0"
                        n2636 = call "Monta Comando.vi"("Set Point"=" A0 20", "Comando"="ESCREVER", "Dispositivo"="TAMPAS" ("Comando"), "Controlador"=w3235) -> ("Resposta"=w3229:string)  [unwired: 1 in, 4 out]
                        n2637 = Tick Count (ms)() -> (millisecond timer value=→"T2":u32)
                        n2638 = Not Equal?(x=w3229, y="TAMPAS OK") -> ()  [unwired: 1 out]
                        n2639 = Select(t="REPOUSO" ("y"), s=FALSE, f="ESPERA 2") -> (s? t:f=w3230:string)
                      }
                      frame "ESPERA 2" {
                        # "25 SEGUNDOS"
                        n2640 = local read "T2"() -> (w3241:u32)
                        n2641 = Tick Count (ms)() -> (millisecond timer value=w3239:u32)
                        n2642 = Add(x=w3241, y=u32 25000) -> (x+y=w3238:u32)
                        n2643 = Greater?(x=w3239, y=w3238) -> (0:w3236:bool)
                        n2644 = case shown="True" w3236 {
                          frame False {
                          }
                          frame True {
                            n2645 = local write "LED ACTION"(TRUE ("LED ACTION")) -> ()
                          }
                        }
                        n2646 = Select(t="REPOUSO" ("y"), s=w3236, f="ESPERA 2" ("y")) -> (s? t:f=w3237:string)
                      }
                      frame "REPOUSO" {
                      }
                    }
                    n2647 = local write "ESTADO ABRIR"(w3203) -> ()
                  }
                  frame True {
                    # "NOVO"
                    # "ABRIR"
                    # "FECHAR"
                    n2648 = local read "ESTADO FECHAR"() -> (w3318:string)
                    n2649 = case shown="\"PIZZA3\"" w3318 {
                      tunnel: [w3383 w3391 w3402 w3410 w3418 "REPOUSO" ("y")] -> w3317
                      frame "INICIO", Default {
                        w3388 = u16 3 items=["ZERO", "AH", "DEC", "TUBO", "CUP"] ("Controlador")
                        # "SELECIONA DISPOSITVO BACIA E\nMANDA FECHAR"
                        n2650 = call "Monta Comando.vi"("Set Point"=" A0 A0", "Comando"="ESCREVER", "Dispositivo"="TAMPAS" ("Comando"), "Controlador"=w3388) -> ("Resposta"=w3384:string)  [unwired: 1 in, 4 out]
                        n2651 = Not Equal?(x=w3384, y="TAMPAS OK") -> ()  [unwired: 1 out]
                        n2652 = Tick Count (ms)() -> (millisecond timer value=→"TF1":u32)
                        n2653 = Select(t="REPOUSO" ("y"), s=FALSE, f="ESPERA1" ("y")) -> (s? t:f=w3383:string)
                      }
                      frame "ESPERA1" {
                        # "20 SEGUNDOS"
                        n2654 = local read "TF1"() -> (w3396:u32)
                        n2655 = Tick Count (ms)() -> (millisecond timer value=w3394:u32)
                        n2656 = Add(x=w3396, y=u32 20000) -> (x+y=w3393:u32)
                        n2657 = Greater?(x=w3394, y=w3393) -> (0:w3390:bool)
                        n2658 = Select(t="PIZZA" ("y"), s=w3390, f="ESPERA1" ("y")) -> (s? t:f=w3391:string)
                      }
                      frame "PIZZA" {
                        w3407 = u16 3 items=["ZERO", "AH", "DEC", "TUBO", "CUP"] ("Controlador")
                        # "PASSA PARA MODO\nHANDSET E PIZZA FECHA"
                        n2659 = call "Monta Comando.vi"("Set Point"=" 48 00", "Comando"="ESCREVER", "Dispositivo"="TAMPAS" ("Comando"), "Controlador"=w3407) -> ("Resposta"=w3401:string)  [unwired: 1 in, 4 out]
                        n2660 = Tick Count (ms)() -> (millisecond timer value=→"TF2":u32)
                        n2661 = Not Equal?(x=w3401, y="TAMPAS OK") -> ()  [unwired: 1 out]
                        n2662 = Select(t="REPOUSO" ("y"), s=FALSE, f="ESPERA2") -> (s? t:f=w3402:string)
                      }
                      frame "ESPERA2" {
                        # "10 SEGUNDOS"
                        n2663 = local read "TF2"() -> (w3408:u32)
                        n2664 = Tick Count (ms)() -> (millisecond timer value=w3414:u32)
                        n2665 = Add(x=w3408, y=u32 10000) -> (x+y=w3415:u32)
                        n2666 = Greater?(x=w3414, y=w3415) -> (0:w3409:bool)
                        n2667 = Select(t="PIZZA3" ("y"), s=w3409, f="ESPERA2" ("y")) -> (s? t:f=w3410:string)
                      }
                      frame "PIZZA3" {
                        w3426 = u16 3 items=["ZERO", "AH", "DEC", "TUBO", "CUP"] ("Controlador")
                        n2668 = call "Monta Comando.vi"("Set Point"=" 48 48", "Comando"="ESCREVER", "Dispositivo"="TAMPAS" ("Comando"), "Controlador"=w3426) -> ("Resposta"=w3421:string)  [unwired: 1 in, 4 out]
                        n2669 = case shown="True" "Case Constant\n(See Context Help) 12" {
                          frame False {
                          }
                          frame True {
                            n2670 = local write "LED ACTION"(FALSE ("LED ACTION")) -> ()
                          }
                        }
                        n2671 = Not Equal?(x=w3421, y="TAMPAS OK") -> ()  [unwired: 1 out]
                        n2672 = Select(t="REPOUSO" ("y"), s=FALSE, f="REPOUSO" ("y")) -> (s? t:f=w3418:string)
                      }
                      frame "REPOUSO" {
                      }
                    }
                    n2673 = local write "ESTADO FECHAR"(w3317) -> ()
                    n2674 = local read "ESTADO ABRIR"() -> (w3316:string)
                    n2675 = case shown="\"ESPERA3\"" w3316 {
                      tunnel: [w3323 w3331 w3339 w3349 w3358 w3371 "REPOUSO" ("y")] -> w3315
                      frame "INICIO", Default {
                        w3329 = u16 3 items=["ZERO", "AH", "DEC", "TUBO", "CUP"] ("Controlador")
                        # "PASSA PARA MODO HANDSET"
                        n2676 = call "Monta Comando.vi"("Set Point"=" F8 00", "Comando"="ESCREVER", "Dispositivo"="TAMPAS" ("Comando"), "Controlador"=w3329) -> ("Resposta"=w3324:string)  [unwired: 1 in, 4 out]
                        n2677 = Not Equal?(x=w3324, y="TAMPAS OK") -> ()  [unwired: 1 out]
                        n2678 = Tick Count (ms)() -> (millisecond timer value=→"TA1":u32)
                        n2679 = Select(t="REPOUSO" ("y"), s=FALSE, f="ESPERA1" ("y")) -> (s? t:f=w3323:string)
                      }
                      frame "ESPERA1" {
                        # "1 SEGUNDO"
                        n2680 = local read "TA1"() -> (w3330:u32)
                        n2681 = Tick Count (ms)() -> (millisecond timer value=w3336:u32)
                        n2682 = Add(x=w3330, y=u32 1000) -> (x+y=w3335:u32)
                        n2683 = Greater?(x=w3336, y=w3335) -> (0:w3333:bool)
                        n2684 = Select(t="ABREPIZZA" ("y"), s=w3333, f="ESPERA1" ("y")) -> (s? t:f=w3331:string)
                      }
                      frame "ABREPIZZA" {
                        w3348 = u16 3 items=["ZERO", "AH", "DEC", "TUBO", "CUP"] ("Controlador")
                        # "MANDA PIZZA ABRIR"
                        n2685 = call "Monta Comando.vi"("Set Point"=" 48 48", "Comando"="ESCREVER", "Dispositivo"="TAMPAS" ("Comando"), "Controlador"=w3348) -> ("Resposta"=w3343:string)  [unwired: 1 in, 4 out]
                        n2686 = Not Equal?(x=w3343, y="TAMPAS OK") -> ()  [unwired: 1 out]
                        n2687 = Tick Count (ms)() -> (millisecond timer value=→"TA2":u32)
                        n2688 = Select(t="ABREPIZZA" ("y"), s=FALSE, f="ESPERA2" ("y")) -> (s? t:f=w3339:string)
                      }
                      frame "ESPERA2" {
                        # "10 SEGUNDOS"
                        n2689 = local read "TA2"() -> (w3350:u32)
                        n2690 = Tick Count (ms)() -> (millisecond timer value=w3355:u32)
                        n2691 = Add(x=w3350, y=u32 10000) -> (x+y=w3354:u32)
                        n2692 = Greater?(x=w3355, y=w3354) -> (0:w3352:bool)
                        n2693 = Select(t="BACIAABRINDO" ("y"), s=w3352, f="ESPERA2" ("y")) -> (s? t:f=w3349:string)
                      }
                      frame "BACIAABRINDO" {
                        w3367 = u16 3 items=["ZERO", "AH", "DEC", "TUBO", "CUP"] ("Controlador")
                        # "BACIA ABRINDO"
                        n2694 = call "Monta Comando.vi"("Set Point"=" A0 20", "Comando"="ESCREVER", "Dispositivo"="TAMPAS" ("Comando"), "Controlador"=w3367) -> ("Resposta"=w3362:string)  [unwired: 1 in, 4 out]
                        n2695 = Not Equal?(x=w3362, y="TAMPAS OK") -> ()  [unwired: 1 out]
                        n2696 = Tick Count (ms)() -> (millisecond timer value=→"TA3":u32)
                        n2697 = Select(t="BACIAABRINDO" ("y"), s=FALSE, f="ESPERA3" ("y")) -> (s? t:f=w3358:string)
                      }
                      frame "ESPERA3" {
                        # "25 SEGUNDOS"
                        n2698 = local read "TA3"() -> (w3369:u32)
                        n2699 = Tick Count (ms)() -> (millisecond timer value=w3374:u32)
                        n2700 = Add(x=w3369, y=u32 25000) -> (x+y=w3373:u32)
                        n2701 = Greater?(x=w3374, y=w3373) -> (0:w3368:bool)
                        n2702 = case shown="True" w3368 {
                          frame False {
                          }
                          frame True {
                            n2703 = local write "LED ACTION"(TRUE ("LED ACTION")) -> ()
                          }
                        }
                        n2704 = Select(t="REPOUSO" ("y"), s=w3368, f="ESPERA3" ("y")) -> (s? t:f=w3371:string)
                      }
                      frame "REPOUSO" {
                      }
                    }
                    n2705 = local write "ESTADO ABRIR"(w3315) -> ()
                  }
                }
              }
              frame #2 {
                # "MÁQUINA DE ESTADOS PROTEÇÃO"
                n2706 = case shown="3" "M_PROT" {
                  selector: "M_PROT" -> [w3432 _ _ _ _ _]
                  tunnel: [w3432 w3433 w3452 5 5 ("estadoCUP") 0 ("estadoCUP")] -> w3430
                  frame 0, Default {
                    # "Sem movimento"
                    n2707 = call "TickTimeout.vi"() -> ("msTick"=→"Timeout PROT":u32)  [unwired: 2 in, 2 out]
                  }
                  frame 1 {
                    w3436 = u16 3 items=["Alarme", "Atencao", "Erro", "Ocupado", "Protecao", "Embreagem", "Tracking", "Var. Track", "Rápido", "Ligeiro", "Médio", "Lento", "Em movimento", ""] ("NomeStatus")
                    w3435 = u16 3 items=["Alarme", "Atencao", "Erro", "Ocupado", "Protecao", "Embreagem", "Tracking", "Var. Track", "Rápido", "Ligeiro", "Médio", "Lento", "Em movimento", ""] ("NomeStatus")
                    # "Testa Ocupado"
                    n2708 = call "Bit Status DEC.vi"("NomeStatus"=w3435) -> ("StatBit"=w3437:bool)
                    n2709 = call "Bit Status AH.vi"("NomeStatus"=w3436) -> ("StatBit"=w3438:bool)
                    n2710 = Or(x=w3438, y=w3437) -> (x .or. y?=w3434:bool)
                    n2711 = case shown="False" w3434 {
                      tunnel: [2 w3449] -> w3433
                      frame False {
                        w3445 = u16 2 items=["ZERO", "AH", "DEC", "TUBO", "CUP"] ("Controlador")
                        w3440 = u16 1 items=["ZERO", "AH", "DEC", "TUBO", "CUP"] ("Controlador")
                        # "Comando para os controladores\nsaírem da Proteção"
                        n2712 = call "Monta Comando.vi"("Comando"="LIBERAR", "Dispositivo"="EIXO" ("Comando"), "Controlador"=w3440) -> ()  [unwired: 2 in, 5 out]
                        n2713 = call "Monta Comando.vi"("Comando"="LIBERAR", "Dispositivo"="EIXO" ("Comando"), "Controlador"=w3445) -> ()  [unwired: 2 in, 5 out]
                      }
                      frame True {
                        # "Busy"
                        n2714 = local read "Timeout PROT"() -> (w3448:u32)
                        n2715 = call "TickTimeout.vi"("msInicial"=w3448, "msTimeout"=u32 20000) -> ("Timeout"=w3446:bool)  [unwired: 2 out]
                        n2716 = case shown="False" w3446 {
                          tunnel: [1 3] -> w3449
                          frame False {
                          }
                          frame True {
                          }
                        }
                      }
                    }
                  }
                  frame 2 {
                    # "Cálculos rápidos"
                    # "Vem do Setup"
                    # "Aguarda Sair da proteção"
                    n2717 = global read "Global_Telescopio.vi" "Zenital angle GRAUS"() -> (w3455:dbl)
                    n2718 = global read "Global_Telescopio.vi" "Z_LIBERA_GRAUS"() -> (w3454:dbl)
                    n2719 = Less?(x=w3455, y=w3454) -> (x < y?=w3453:bool)
                    n2720 = case shown="True" w3453 {
                      tunnel: [2 ("estadoCUP") 4 ("estadoCUP")] -> w3452
                      frame False {
